vi "获取根目录下所有保存图片文件路径.vi"() -> (1 "图片张数":i32, 2 "所有图片路径":path[](array[path]))   [LabVIEW 2014]
uses:
  Global.vi
panel:
  out "路径输出":path
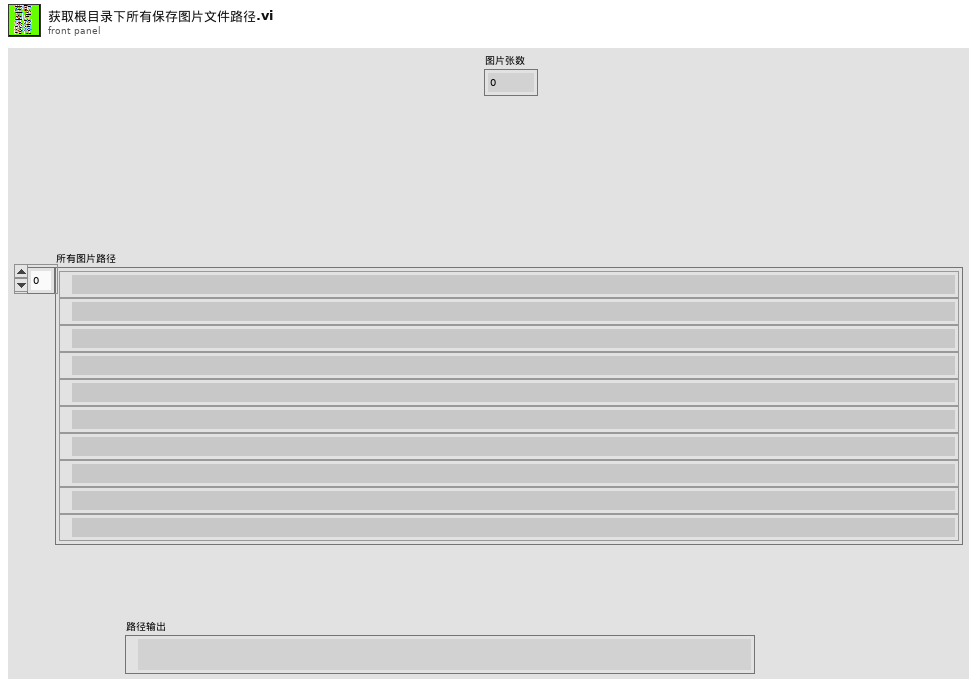
[diagram p1: front panel]
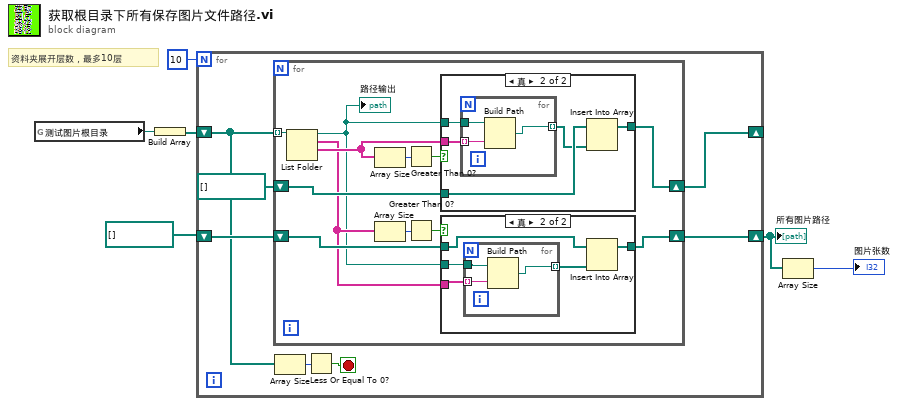
[diagram p0: block diagram]
diagram:
  # "资料夹展开层数，最多10层"
  n1 = global read "Global.vi" "测试图片根目录"() -> (w6:path)
  n2 = Build Array(w6) -> (w5:path[])
  n3 = for {
    N: 10 -> [_]
    shift-right: [w12] -> _
    shift-left: w5 -> [w8]
    shift-right: [w11] -> w2
    shift-left: path[] [] -> [w10]
    stop <- w7 stop-if-true
    n4 = for {
      tunnel: w8 -> [w25] mode=indexing
      shift-right: [w23] -> w12
      shift-left: path[] [] -> [w24]
      shift-right: [w15] -> w11
      shift-left: w10 -> [w19]
      n5 = List Folder ("罗列文件夹")(path=w25) -> (path out=w14:path, filenames=w16:string[], folder names=w20:string[])  [unwired: 3 in, 1 out]
      "路径输出" <- w14
      n6 = Array Size(array=w20) -> (size(s)=w22:i32)
      n7 = Array Size(array=w16) -> (size(s)=w18:i32)
      n8 = Greater Than 0?(x=w22) -> (x > 0?=w21:bool)
      n9 = Greater Than 0?(x=w18) -> (x > 0?=w17:bool)
      n10 = case shown="真" w21 {
        tunnel: w14 -> [_ w40]
        tunnel: w20 -> [_ w39]
        tunnel: [w35 w38] -> w23
        tunnel: w24 -> [w35 w37]
        frame False {
        }
        frame True {
          n11 = for {
            tunnel: w40 -> [w43]
            tunnel: w39 -> [w42] mode=indexing
            tunnel: [w41] -> w36 mode=indexing
            n12 = Build Path(base path=w43, name or relative path=w42) -> (appended path=w41:path)
          }
          n13 = Insert Into Array(array=w37, new element=w36) -> (w38:path[])  [unwired: 1 in]
        }
      }
      n14 = case shown="真" w17 {
        tunnel: w19 -> [w26 w29]
        tunnel: [w26 w31] -> w15
        tunnel: w16 -> [_ w30]
        tunnel: w14 -> [_ w27]
        frame False {
        }
        frame True {
          n15 = for {
            tunnel: w30 -> [w34] mode=indexing
            tunnel: [w33] -> w28 mode=indexing
            tunnel: w27 -> [w32]
            n16 = Build Path(base path=w32, name or relative path=w34) -> (appended path=w33:path)
          }
          n17 = Insert Into Array(array=w29, new element=w28) -> (w31:path[])  [unwired: 1 in]
        }
      }
    }
    n18 = Array Size(array=w8) -> (size(s)=w9:i32)
    n19 = Less Or Equal To 0?(x=w9) -> (x <= 0?=w7:bool)
  }
  "所有图片路径" <- w2
  n20 = Array Size(array=w2) -> (size(s)=→"图片张数":i32)
